vi "Read T (ms).vi"(11 "State in":refnum<class "State.lvclass">) -> (2 "T (ms)":u32, 3 "State out":refnum<class "State.lvclass">)   [LabVIEW 2019, in "Userlib.lvlib" / "State.lvclass"]
uses:
  State.lvclass
  State.lvclass/State.ctl
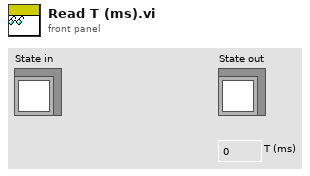
[diagram p1: front panel]
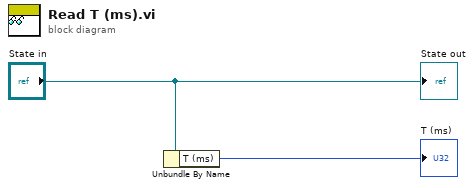
[diagram p0: block diagram]
diagram:
  n1 = Unbundle By Name("State in") -> ("T (ms)"=→"T (ms)":u32)
  "State out" <- "State in"
